vi "Implement IIR Direct Filter (DBL).vi"(0 "signal in":waveform(dbl)={"t0"=timestamp(2.7999999999999994 s since 1904-01-01), "dt"=0.001, "Y"=[]}, 1 "reverse coefficients":dbl[](array[numeric]) format="%0.2f", 2 "forward coefficients":dbl[](array[numeric]) format="%0.2f", 3 "error in (no error)":errorcluster, 4 "reset filter":bool) -> (5 "signal out":waveform(dbl), 6 "error out":errorcluster)   [LabVIEW 2020, in "NI_MAPro.lvlib"]
uses:
  NI_MAPro.lvlib
  NI_MABase.lvlib
  NI_AALBase.lvlib
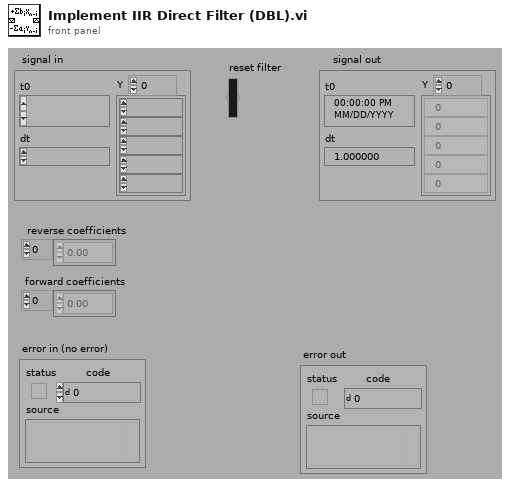
[diagram p1: front panel]
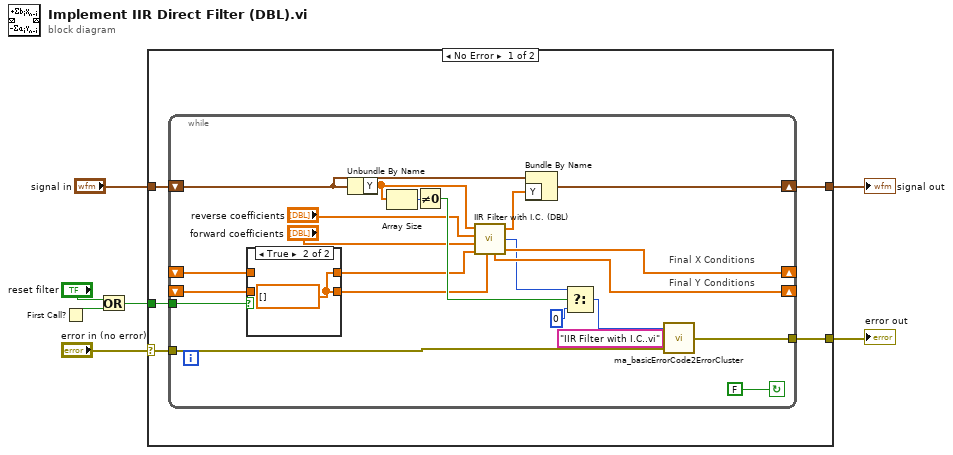
[diagram p0: block diagram]
diagram:
  n1 = First Call?() -> (First Call?: T/F=w4:bool)
  n2 = Or(x="reset filter", y=w4) -> (x .or. y?=w3:bool)
  n3 = case shown="No Error" "error in (no error)" {
    selector: "error in (no error)" -> [w10 w39]
    tunnel: [w12 w39] -> w6
    tunnel: w3 -> [w11 _]
    tunnel: "signal in" -> [w9 w38]
    tunnel: [w8 w38] -> w1
    frame No Error {
      n4 = while {
        tunnel: w10 -> [w19]
        tunnel: w11 -> [w21]
        tunnel: [w25] -> w12
        shift-left: w9 -> [w22]
        shift-right: [w24] -> w8
        shift-left: _ -> [w28]
        shift-right: [w30] -> _
        shift-left: _ -> [w26]
        shift-right: [w31] -> _
        stop <- FALSE continue-if-true
        # "Final Y Conditions"
        # "Final X Conditions"
        n5 = case shown="True" w21 {
          tunnel: w28 -> [w36 _]
          tunnel: [w36 w37] -> w29
          tunnel: w26 -> [w35 _]
          tunnel: [w35 w37] -> w27
          frame False {
          }
          frame True {
            w37 = dbl[] [] ("Final X Conditions")
          }
        }
        n6 = Unbundle By Name(w22) -> ("Y"=w13:dbl[])
        n7 = Array Size(array=w13) -> (size(s)=w14:i32)
        n8 = Not Equal To 0?(x=w14) -> (x != 0?=w34:bool)
        n9 = call "IIR Filter with I.C. (DBL).vi"("Initial Y Conditions"=w29, "Initial X Conditions"=w27, "Forward Coefficients"="forward coefficients", "Reverse Coefficients"="reverse coefficients", "X"=w13) -> ("Final X Conditions"=w31:dbl[], "Final Y Conditions"=w30:dbl[], "error"=w16:i32, "Filtered X"=w20:dbl[])  [unwired: 2 in]
        n10 = Bundle By Name(cluster=w22, "Y"=w20) -> (w24:waveform(dbl))
        n11 = Select(t=w16, s=w34, f=0) -> (s? t:f=w15:i32)
        n12 = call "ma_basicErrorCode2ErrorCluster.vi"("error in (no error)"=w19, "subVI name"="IIR Filter with I.C..vi", "Error Code"=w15) -> ("error out"=w25:errorcluster)
      }
    }
    frame Error {
    }
  }
  "error out" <- w6
  "signal out" <- w1
